vi "Servo MSMT Set Servo Type in Measurement Name.vi"(8 "error in (no error)":errorcluster, 11 "Servo MSMT in":refnum<class "Servo MSMT.lvclass">) -> (0 "error out":errorcluster, 3 "Servo MSMT out":refnum<class "Servo MSMT.lvclass">)   [LabVIEW 2018, in "Servo MSMT.lvlib" / "Servo MSMT.lvclass"]
uses:
  Servo MSMT.lvclass
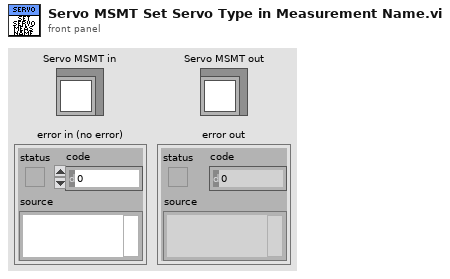
[diagram p1: front panel]
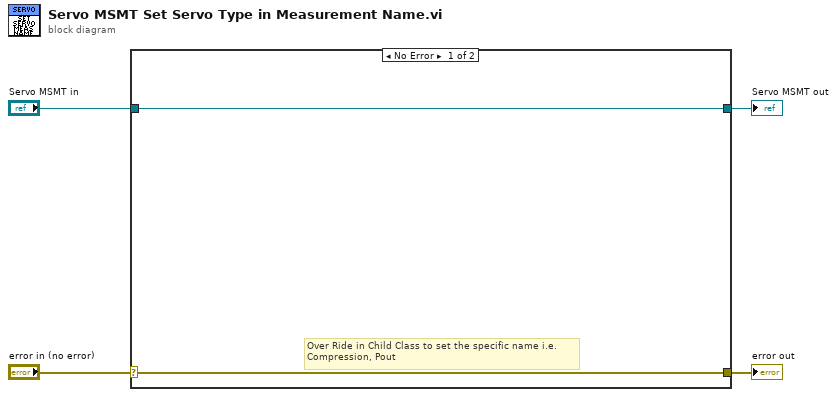
[diagram p0: block diagram]
diagram:
  n1 = case shown="No Error" "error in (no error)" {
    selector: "error in (no error)" -> [w5 w8]
    tunnel: [w5 w8] -> w3
    tunnel: [w6 w7] -> w1
    tunnel: "Servo MSMT in" -> [w6 w7]
    frame No Error {
      # "Over Ride in Child Class to set the specific name i.e.\nCompression, Pout"
    }
    frame Error {
    }
  }
  "error out" <- w3
  "Servo MSMT out" <- w1
